vi "Bundle RT Configuration.vi"(8 "error in (no error)":errorcluster) -> (0 "error out":errorcluster, 3 "All Control Configuration Values":T1)   [LabVIEW 2022 SP3]
uses:
  controls/All Control Configuration Values.ctl
  controls/Control State.ctl
  controls/Raw Values.ctl
  controls/Control Configuration.ctl
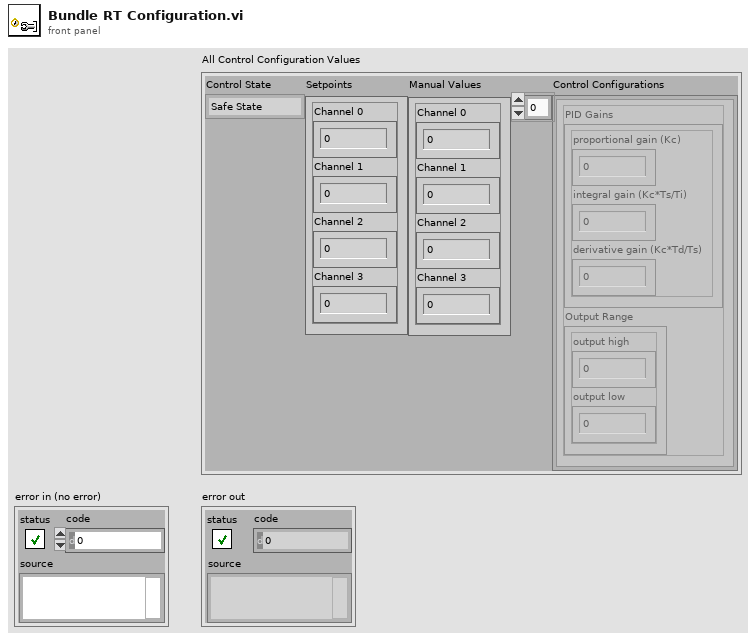
[diagram p1: front panel]
types:
  T1 = typedef "All Control Configuration Values.ctl" = cluster{"Control State":T2, "Setpoints":T3, "Manual Values":T3, "Control Configurations":T4[]}
  T2 = typedef "Control State.ctl" = enum16{"Safe State", "Manual", "Control (PID)"}
  T3 = typedef "Raw Values.ctl" = cluster{"Channel 0":dbl, "Channel 1":dbl, "Channel 2":dbl, "Channel 3":dbl}
  T4 = typedef "Control Configuration.ctl" = cluster{"PID Gains":cluster{"proportional gain (Kc)":dbl, "integral gain (Kc*Ts/Ti)":dbl, "derivative gain (Kc*Td/Ts)":dbl}, "Output Range":cluster{"output high":dbl, "output low":dbl}}
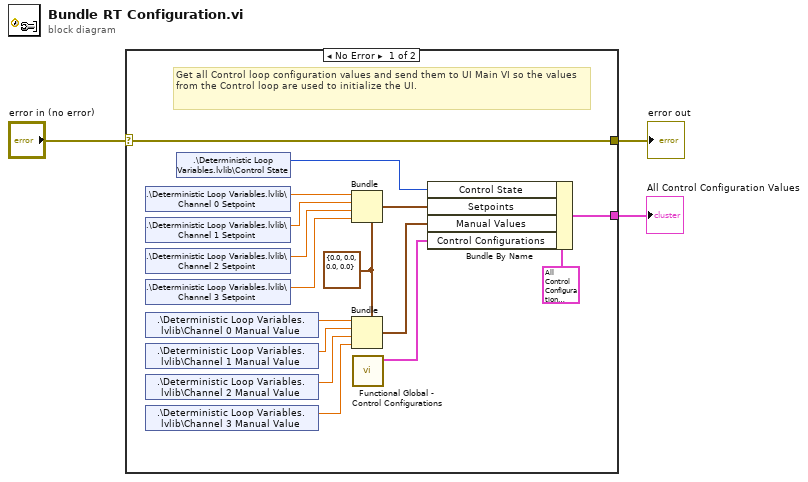
[diagram p0: block diagram]
diagram:
  n1 = case shown="No Error" "error in (no error)" {
    selector: "error in (no error)" -> [w17 w20]
    tunnel: [w17 w20] -> w2
    tunnel: [w18 _] -> w1
    frame No Error {
      w5 = T3 {"Channel 0"=0.0, "Channel 1"=0.0, "Channel 2"=0.0, "Channel 3"=0.0} ("Raw Values")
      # "Get all Control loop configuration values and send them to UI Main VI so the values from the Control loop are used to initialize the UI."
      n2 = shared-variable ".\\Deterministic Loop Variables.lvlib\\Channel 0 Setpoint"() -> (w13:dbl)  [unwired: 1 in, 1 out]
      n3 = shared-variable ".\\Deterministic Loop Variables.lvlib\\Channel 1 Setpoint"() -> (w12:dbl)  [unwired: 1 in, 1 out]
      n4 = shared-variable ".\\Deterministic Loop Variables.lvlib\\Channel 2 Setpoint"() -> (w11:dbl)  [unwired: 1 in, 1 out]
      n5 = shared-variable ".\\Deterministic Loop Variables.lvlib\\Channel 3 Setpoint"() -> (w10:dbl)  [unwired: 1 in, 1 out]
      n6 = shared-variable ".\\Deterministic Loop Variables.lvlib\\Channel 0 Manual Value"() -> (w6:dbl)  [unwired: 1 in, 1 out]
      n7 = shared-variable ".\\Deterministic Loop Variables.lvlib\\Channel 1 Manual Value"() -> (w7:dbl)  [unwired: 1 in, 1 out]
      n8 = shared-variable ".\\Deterministic Loop Variables.lvlib\\Channel 2 Manual Value"() -> (w8:dbl)  [unwired: 1 in, 1 out]
      n9 = shared-variable ".\\Deterministic Loop Variables.lvlib\\Channel 3 Manual Value"() -> (w9:dbl)  [unwired: 1 in, 1 out]
      n10 = shared-variable ".\\Deterministic Loop Variables.lvlib\\Control State"() -> (w14:T2)  [unwired: 1 in, 1 out]
      n11 = Bundle(cluster=w5, "Channel 0"=w13, "Channel 1"=w12, "Channel 2"=w11, "Channel 3"=w10) -> (w16:T3)
      n12 = Bundle(cluster=w5, "Channel 0"=w6, "Channel 1"=w7, "Channel 2"=w8, "Channel 3"=w9) -> (w4:T3)
      n13 = call "Functional Global - Control Configurations.vi"() -> ("Control Configurations out"=w15:T4[])  [unwired: 11 in]
      n14 = Bundle By Name(cluster=T1 {"Control State"=enum."Safe State", "Setpoints"={"Channel 0"=0.0, "Channel 1"=0.0, "Channel 2"=0.0, "Channel 3"=0.0}, "Manual Values"={"Channel 0"=0.0, "Channel 1"=0.0, "Channel 2"=0.0, "Channel 3"=0.0}, "Control Configurations"=[]} ("All FPGA Configuration Values"), "Control State"=w14, "Setpoints"=w16, "Manual Values"=w4, "Control Configurations"=w15) -> (w18:T1)
    }
    frame Error {
    }
  }
  "error out" <- w2
  "All Control Configuration Values" <- w1
